vi "Write Rate.vi"(8 "error in (no error)":errorcluster, 10 "Rate":dbl, 11 "AInterestAccount in":refnum<class "AInterestAccount.lvclass">) -> (0 "error out":errorcluster, 3 "AInterestAccount out":refnum<class "AInterestAccount.lvclass">)   [LabVIEW 2020, in "AInterestAccount.lvclass"]
uses:
  AInterestAccount.lvclass
  AInterestAccount.lvclass/AInterestAccount.ctl
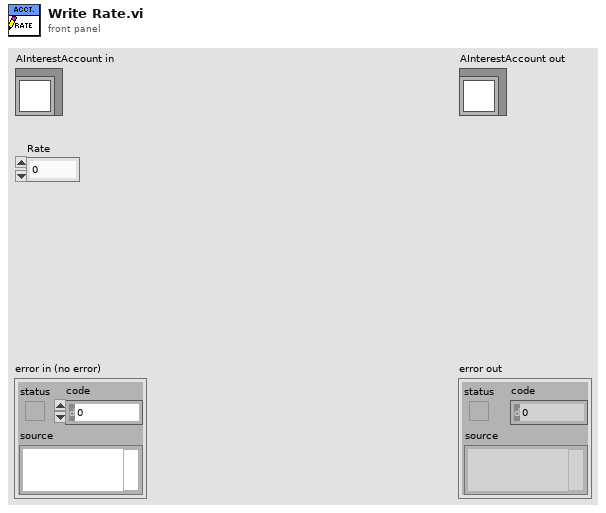
[diagram p1: front panel]
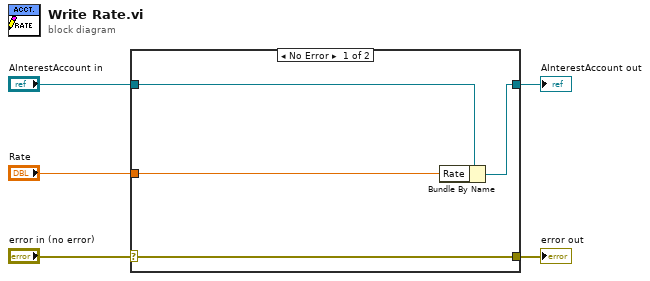
[diagram p0: block diagram]
diagram:
  n1 = case shown="No Error" "error in (no error)" {
    selector: "error in (no error)" -> [w9 w10]
    tunnel: [w9 w10] -> w4
    tunnel: [w7 w11] -> w2
    tunnel: "AInterestAccount in" -> [w8 w11]
    tunnel: "Rate" -> [w6 _]
    frame No Error {
      n2 = Bundle By Name(cluster=w8, "Rate"=w6) -> (w7:refnum<class "AInterestAccount.lvclass">)
    }
    frame Error {
    }
  }
  "error out" <- w4
  "AInterestAccount out" <- w2
